vi "is a.vi"(8 "error in (no error)":errorcluster, 11 "PXI 4110 in":refnum<class "PXI 4110.lvclass">) -> (0 "error out":errorcluster, 2 "is a":string, 3 "PXI 4110 out":refnum<class "PXI 4110.lvclass">)   [LabVIEW 2017, in "PXI 4110.lvclass"]
uses:
  PXI 4110.lvclass
  MAL-Framework/user.lib/Common Components/Hardware/PSU/PSU.lvclass
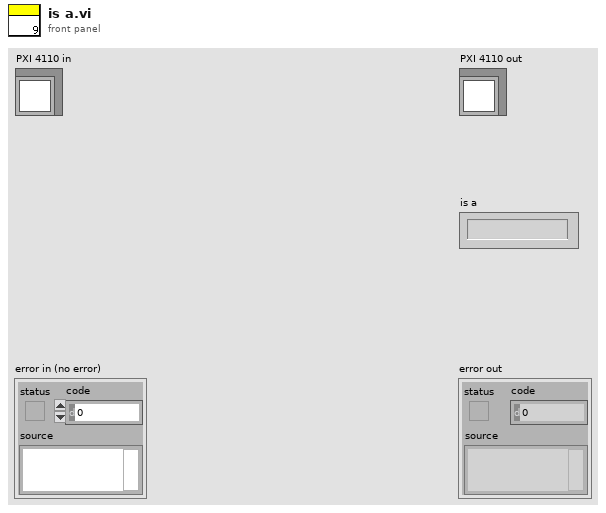
[diagram p1: front panel]
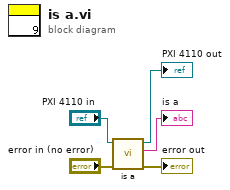
[diagram p0: block diagram]
diagram:
  n1 = call-parent "is a.vi"("error in (no error)"="error in (no error)", "PSU in"="PXI 4110 in") -> ("error out"=→"error out":errorcluster, "is a"=→"is a":string, "PSU out"=→"PXI 4110 out":refnum<class "PXI 4110.lvclass">)  [unwired: 7 in]
